vi "TD of String.vi"() -> ()   [LabVIEW 2012, in "TD Tools.lvlib"]
uses:
  TD Tools.lvlib
panel:
  out "数据字符串":string
  out "类型字符串":i16[](array[numeric]) format="dec:%d\nhex:%04x"
  in  "Str":string
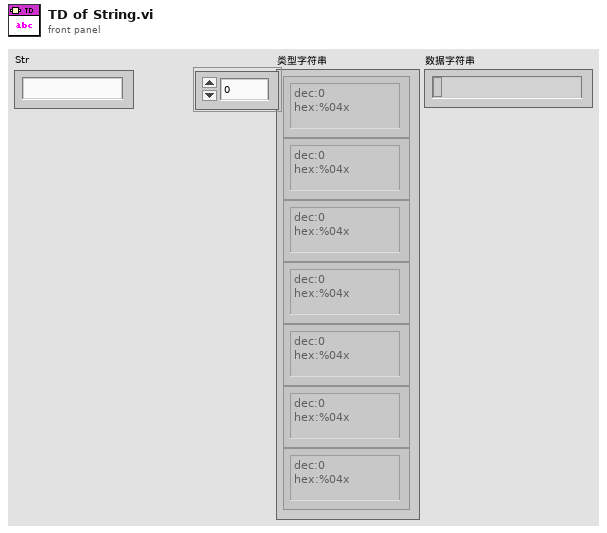
[diagram p1: front panel]
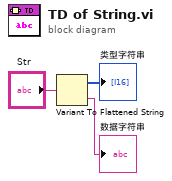
[diagram p0: block diagram]
diagram:
  n1 = Variant To Flattened String(Variant="Str") -> (data string=→"数据字符串":string, 1:→"类型字符串":i16[])
